vi "HH Config.vi"(8 "Device Inputs":dbl[](array[numeric]), 10 "FIFO Indexes.Write.HH Config":T1[](array[typedef]) {"ISeq"."Duration [s]" min=0 max=26; "ISeq"."Lower [A]" min=0 max=8; "ISeq"."Upper [A]" min=0 max=8}) -> (3 "HH Config":T2[](array[typedef]) {"ISeq"."Duration [s]" min=0 max=26 format="%#_3p"; "ISeq"."Lower [A]" min=0 max=8 format="%#_3p"; "ISeq"."Upper [A]" min=0 max=8 format="%#_3p"})   [LabVIEW 2016, in "DCM Engine.lvlib"]
uses:
  DCM Engine.lvlib
  Built/DCM Classes Packed/Pharlap/C/DCM-Classes.lvlibp/DCM/HH/RT/Config.ctl
  Built/DCM Classes Packed/Pharlap/C/DCM-Classes.lvlibp/DCM/HH/RT/Mode.ctl
  Built/DCM Classes Packed/Pharlap/C/DCM-Classes.lvlibp/DCM/HH/RT/ISeq.ctl
  Shared/Types/HH Config Indexes.ctl
  Built/DCM Classes Packed/Pharlap/C/DCM-Classes.lvlibp/DCM/HH/RT/DCM - RT - HH.lvlib
  DCM Shared.lvlib
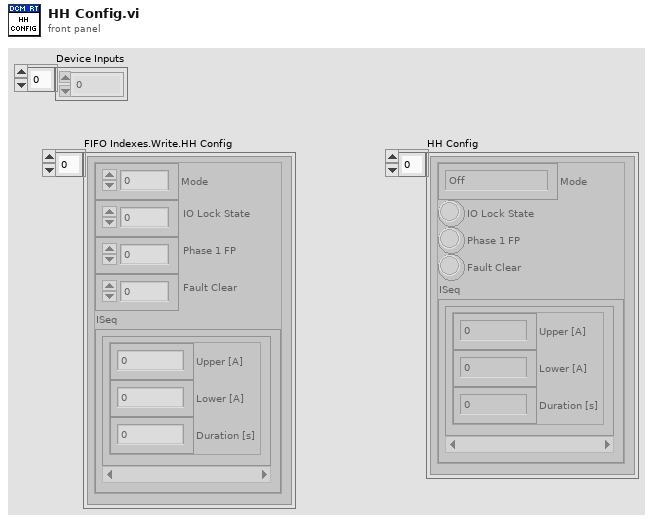
[diagram p1: front panel]
types:
  T1 = typedef "DCM Shared.lvlib/HH Config Indexes.ctl" = cluster{"Mode":i32, "IO Lock State":i32, "Phase 1 FP":i32, "Fault Clear":i32, "ISeq":cluster{"Upper [A]":i32, "Lower [A]":i32, "Duration [s]":i32}[]}
  T2 = typedef "DCM-Classes.lvlibp/DCM - RT - HH.lvlib/Config.ctl" = cluster{"Mode":T3, "IO Lock State":bool, "Phase 1 FP":bool, "Fault Clear":bool, "ISeq":T4[]}
  T3 = typedef "DCM-Classes.lvlibp/DCM - RT - HH.lvlib/Mode.ctl" = enum16{"Off", "Lowside", "Highside", "PFI", "Full H", "3-Phase"}
  T4 = typedef "DCM-Classes.lvlibp/DCM - RT - HH.lvlib/ISeq.ctl" = cluster{"Upper [A]":sgl, "Lower [A]":sgl, "Duration [s]":sgl}
  T5 = cluster{"Upper [A]":i32, "Lower [A]":i32, "Duration [s]":i32}[]
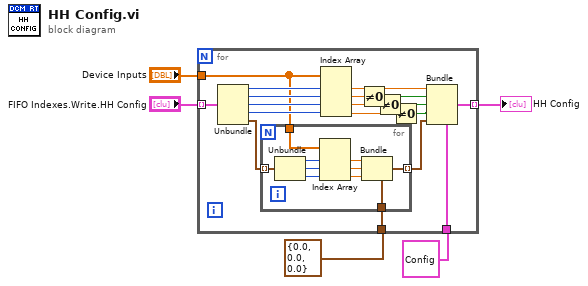
[diagram p0: block diagram]
diagram:
  n1 = for {
    tunnel: "FIFO Indexes.Write.HH Config" -> [w23] mode=indexing
    tunnel: "Device Inputs" -> [w16]
    tunnel: [w18] -> w4 mode=indexing
    tunnel: T4 {"Upper [A]"=0.0, "Lower [A]"=0.0, "Duration [s]"=0.0} -> [w15]
    tunnel: T2 {"Mode"=enum."Off", "IO Lock State"=FALSE, "Phase 1 FP"=FALSE, "Fault Clear"=FALSE, "ISeq"=[{"Upper [A]"=0.0, "Lower [A]"=0.0, "Duration [s]"=0.0}, {"Upper [A]"=0.0, "Lower [A]"=0.0, "Duration [s]"=0.0}]} ("HH Config") -> [w14]
    n2 = Unbundle(w23) -> ("Mode"=w22:i32, "IO Lock State"=w21:i32, "Phase 1 FP"=w20:i32, "Fault Clear"=w19:i32, "ISeq"=w17:T5)
    n3 = for {
      tunnel: w17 -> [w33] mode=indexing
      tunnel: w16 -> [w29]
      tunnel: [w25] -> w6 mode=indexing
      tunnel: w15 -> [w24]
      n4 = Unbundle(w33) -> ("Upper [A]"=w32:i32, "Lower [A]"=w31:i32, "Duration [s]"=w30:i32)
      n5 = Index Array(array=w29, index #1=w32, index #2=w31, index #3=w30) -> (element #1=w28:dbl, element #2=w27:dbl, element #3=w26:dbl)
      n6 = Bundle(cluster=w24, "Upper [A]"=w28, "Lower [A]"=w27, "Duration [s]"=w26) -> (w25:T4)
    }
    n7 = Index Array(array=w16, index #1=w22, index #2=w21, index #3=w20, index #4=w19) -> (element #1=w7:dbl, element #2=w13:dbl, element #3=w9:dbl, element #4=w8:dbl)
    n8 = Not Equal To 0?(x=w13) -> (x != 0?=w12:bool)
    n9 = Not Equal To 0?(x=w9) -> (x != 0?=w11:bool)
    n10 = Not Equal To 0?(x=w8) -> (x != 0?=w10:bool)
    n11 = Bundle(cluster=w14, "Mode"=w7, "IO Lock State"=w12, "Phase 1 FP"=w11, "Fault Clear"=w10, "ISeq"=w6) -> (w18:T2)
  }
  "HH Config" <- w4
